vi "Match Multiple Geometric Patterns.vi"() -> ()   [LabVIEW 2014]
doc: "This example demonstrates how to perform multiple template geometric matching in NI Vision. First, three geometric matching templates are learned as a multiple geometric template. Next, the template is applied to a series of test images. This example uses color coded bounding boxes to display the location of geometric template matches and displays the number of instances of each geometric template match found in the test image."
uses:
  <vilib>/vision/Pattern Matching.llb/IMAQ Match Range Setting.ctl
  <vilib>/vision/NI_Vision_Development_Module.lvlib
panel:
  out "Hanger Matches":i32
  out "Plate Matches":i32
  out "Bracket Matches":i32
  in  "Delay (s.)":dbl(slide)=0.496 scale=0.0..2.0
  out "Image":T1(plugin-control)
  in  "Stop":bool
  in  "Hanger Color":u32(colorbox)=3381759
  in  "Plate Color":u32(colorbox)=6618880
  in  "Bracket Color":u32(colorbox)=16711680
  out "Hanger Template":T1(plugin-control)
  out "Plate Template":T1(plugin-control)
  out "Bracket Template":T1(plugin-control)
  # "Overview: Demonstrates how to use geometric matching to locate parts in an image.\nRequirements: NI Vision Development Module\nInstructions: Run the VI."
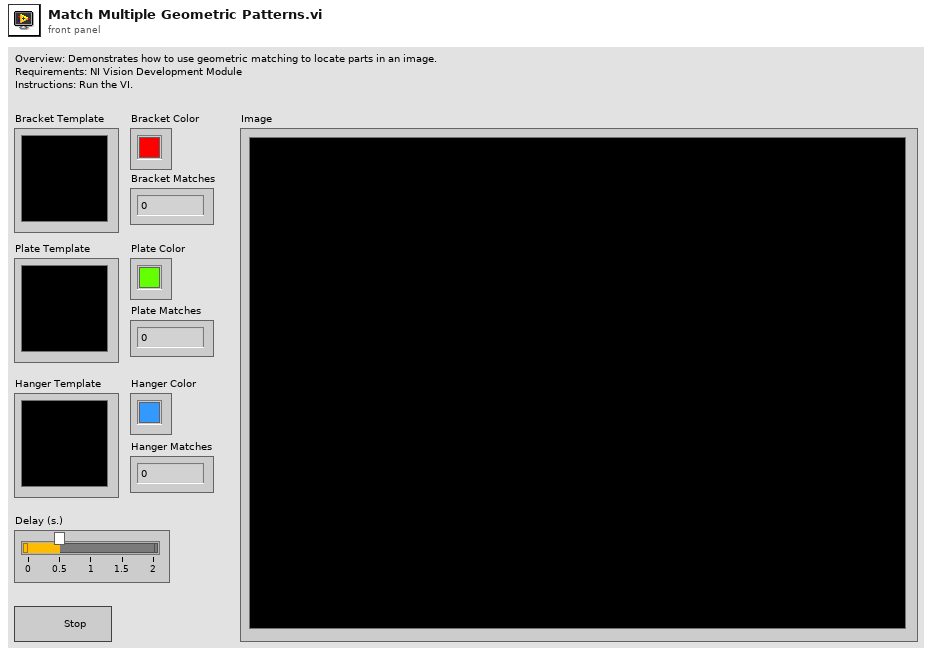
[diagram p1: front panel]
types:
  T1 = typedef "IMAQ Image.ctl" = refnum<image>
  T2 = typedef "IMAQ Match Range Setting.ctl" = cluster{"Match Constraints":u32, "Min":dbl, "Max":dbl}
  T3 = cluster{"Rotation":bool, "Scale":bool, "Occlusion":bool, "Reserved":bool, "Reserved":bool, "Reserved":bool}
  T4 = cluster{"Match Geometric Pattern Setup Data":string, "Number of Matches":i32, "Minimum Match Score":sgl}
  T5 = typedef "IMAQ GM Multiple Template.ctl" = refnum<k20>
  T6 = typedef "IMAQ GM Match Report.ctl" = cluster{"Position":cluster{"x":sgl, "y":sgl}, "Angle":sgl, "Scale":sgl, "Score":sgl, "Bounding Box":cluster{"x":sgl, "y":sgl}[], "Contrast Reversed":bool, "Occlusion %":sgl, "Template Target Curve Score":sgl, "Target Template Curve Score":sgl, "Correlation Score":sgl}
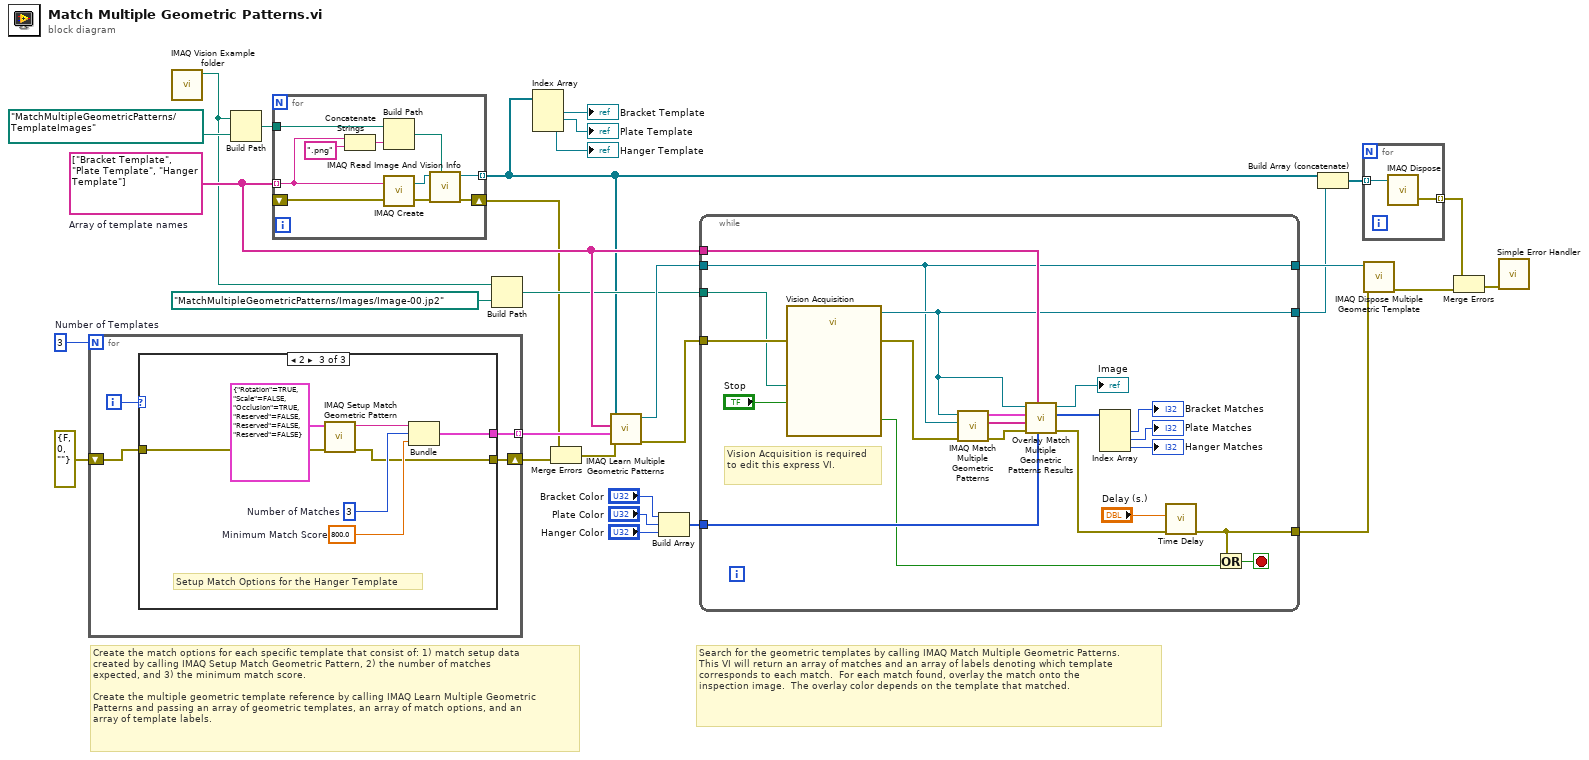
[diagram p0: block diagram]
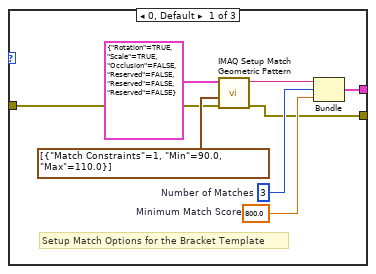
[diagram p2: hidden frame]
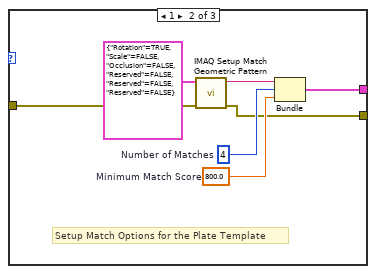
[diagram p3: hidden frame]
diagram:
  w15 = 3  # Number of Templates
  w21 = string[] ["Bracket Template", "Plate Template", "Hanger Template"]  # Array of template names
  # "Search for the geometric templates by calling IMAQ Match Multiple Geometric Patterns.\nThis VI will return an array of matches and an array of labels denoting which template\ncorresponds to each match.  For each match found, overlay the match onto the\ninspection image.  The overlay color depends on the template that matched."
  # "Create the match options for each specific template that consist of: 1) match setup data\ncreated by calling IMAQ Setup Match Geometric Pattern, 2) the number of matches \nexpected, and 3) the minimum match score.\n\nCreate the multiple geometric template reference by calling IMAQ Learn Multiple Geometric\nPatterns and passing an array of geometric templates, an array of match options, and an\narray of template labels."
  n1 = for {
    N: w15 -> [_]
    tunnel: [w33] -> w24 mode=indexing
    shift-right: [w31] -> w10
    shift-left: errorcluster {"status"=FALSE, "code"=0, "source"=""} ("error out") -> [w30]
    i -> [w32]
    n2 = case shown="2" w32 {
      tunnel: [w38 w45 w52] -> w33
      tunnel: [w35 w42 w49] -> w31
      tunnel: w30 -> [w34 w43 w50]
      frame 0, Default {
        w39 = sgl 800.0  # Minimum Match Score
        w40 = 3  # Number of Matches
        # "Setup Match Options for the Bracket Template"
        n3 = call "IMAQ Setup Match Geometric Pattern"("error in (no error)"=w34, "Range Settings"=T2[] [{"Match Constraints"=1, "Min"=90.0, "Max"=110.0}], "Match Mode"=T3 {"Rotation"=TRUE, "Scale"=TRUE, "Occlusion"=FALSE, "Reserved"=FALSE, "Reserved"=FALSE, "Reserved"=FALSE}) -> ("error out"=w35:errorcluster, "Match Geometric Pattern Setup Data"=w41:string)  [unwired: 7 in]
        n4 = Bundle("Match Geometric Pattern Setup Data"=w41, "Number of Matches"=w40, "Minimum Match Score"=w39) -> (w38:T4)  [unwired: 1 in]
      }
      frame 1 {
        w46 = sgl 800.0  # Minimum Match Score
        w47 = 4  # Number of Matches
        # "Setup Match Options for the Plate Template"
        n5 = call "IMAQ Setup Match Geometric Pattern"("error in (no error)"=w43, "Match Mode"=T3 {"Rotation"=TRUE, "Scale"=FALSE, "Occlusion"=FALSE, "Reserved"=FALSE, "Reserved"=FALSE, "Reserved"=FALSE}) -> ("error out"=w42:errorcluster, "Match Geometric Pattern Setup Data"=w48:string)  [unwired: 8 in]
        n6 = Bundle("Match Geometric Pattern Setup Data"=w48, "Number of Matches"=w47, "Minimum Match Score"=w46) -> (w45:T4)  [unwired: 1 in]
      }
      frame 2 {
        w53 = sgl 800.0  # Minimum Match Score
        w54 = 3  # Number of Matches
        # "Setup Match Options for the Hanger Template"
        n7 = call "IMAQ Setup Match Geometric Pattern"("error in (no error)"=w50, "Match Mode"=T3 {"Rotation"=TRUE, "Scale"=FALSE, "Occlusion"=TRUE, "Reserved"=FALSE, "Reserved"=FALSE, "Reserved"=FALSE}) -> ("error out"=w49:errorcluster, "Match Geometric Pattern Setup Data"=w55:string)  [unwired: 8 in]
        n8 = Bundle("Match Geometric Pattern Setup Data"=w55, "Number of Matches"=w54, "Minimum Match Score"=w53) -> (w52:T4)  [unwired: 1 in]
      }
    }
  }
  n9 = call "IMAQ Vision Example folder.vi"() -> ("Example Image Path"=w13:path)  [unwired: 11 in]
  n10 = Build Path(base path=w13, name or relative path=path "MatchMultipleGeometricPatterns/TemplateImages") -> (appended path=w25:path)
  n11 = for {
    tunnel: w21 -> [w61] mode=indexing
    tunnel: w25 -> [w65]
    tunnel: [w62] -> w5 mode=indexing
    shift-right: [w57] -> w9
    shift-left: _ -> [w56]
    n12 = Concatenate Strings(w61, ".png" ("string")) -> (w60:string)
    n13 = Build Path(base path=w65, name or relative path=w60) -> (appended path=w64:path)
    n14 = call "IMAQ Create"("Image Name"=w61, "error in (no error)"=w56) -> ("New Image"=w63:T1, "error out"=w58:errorcluster)  [unwired: 3 in]
    n15 = call "IMAQ Read Image And Vision Info"("File Path"=w64, "error in (no error)"=w58, "Image"=w63) -> ("error out"=w57:errorcluster, "Image Out"=w62:T1)  [unwired: 6 in, 1 out]
  }
  n16 = Build Path(base path=w13, name or relative path=path "MatchMultipleGeometricPatterns/Images/Image-00.jp2") -> (appended path=w12:path)
  n17 = Index Array(array=w5) -> (element #1=→"Bracket Template":T1, element #2=→"Plate Template":T1, element #3=→"Hanger Template":T1)  [unwired: 3 in]
  n18 = Merge Errors(w9, w10) -> (w8:errorcluster)
  n19 = call "IMAQ Learn Multiple Geometric Patterns"("error in (no error)"=w8, "Default Match Options"=w24, "Template Labels"=w21, "Template Images"=w5) -> ("error out"=w20:errorcluster, "Multiple Template (out)"=w23:T5)  [unwired: 6 in]
  n20 = Build Array("Bracket Color", "Plate Color", "Hanger Color") -> (w16:u32[])
  n21 = while {
    tunnel: w23 -> [w67]
    tunnel: w21 -> [w75]
    tunnel: [w67] -> w22
    tunnel: w20 -> [w80]
    tunnel: [w68] -> w6
    tunnel: w16 -> [w73]
    tunnel: w12 -> [w69]
    tunnel: [w66] -> w7
    stop <- w74 stop-if-true
    # "Vision Acquisition is required to edit this express VI."
    n22 = call "Vision Acquisition"("Image Path"=w69, "Stop (F)"="Stop", "error in"=w80) -> ("Image Out"=w68:T1, "Stopped"=w70:bool, "error out"=w72:errorcluster)  [unwired: 22 in]
    n23 = call "IMAQ Match Multiple Geometric Patterns"("error in (no error)"=w72, "Multiple Template"=w67, "Image"=w68) -> ("error out"=w78:errorcluster, "Matched Labels"=w76:string[], "Matches (pixel)"=w77:T6[])  [unwired: 5 in, 1 out]
    n24 = call "Overlay Match Multiple Geometric Patterns Results.vi"("Label Colors"=w73, "Learned Labels"=w75, "error in"=w78, "Match Labels"=w76, "Match Results"=w77, "Image"=w68) -> ("error out"=w71:errorcluster, "Number of Matches"=w79:i32[], "Image Out"=→"Image":T1)  [unwired: 3 in]
    n25 = Index Array(array=w79) -> (element #1=→"Bracket Matches":i32, element #2=→"Plate Matches":i32, element #3=→"Hanger Matches":i32)  [unwired: 3 in]
    n26 = call "Time Delay"("error in (no error)"=w71, "Delay Time (s)"="Delay (s.)") -> ("error out"=w66:errorcluster)  [unwired: 9 in]
    n27 = Or(x=w66, y=w70) -> (x .or. y?=w74:bool)
  }
  n28 = Build Array (concatenate)(w5, w6) -> (w4:T1[])
  n29 = for {
    tunnel: w4 -> [w88] mode=indexing
    tunnel: [w87] -> w2 mode=indexing
    n30 = call "IMAQ Dispose"("Image"=w88) -> ("error out"=w87:errorcluster)  [unwired: 5 in]
  }
  n31 = call "IMAQ Dispose Multiple Geometric Template"("error in (no error)"=w7, "Multiple Template"=w22) -> ("error out"=w3:errorcluster)  [unwired: 9 in]
  n32 = Merge Errors(w2, w3) -> (w1:errorcluster)
  n33 = call <vilib>:"Simple Error Handler.vi"("error in (no error)"=w1) -> ()  [unwired: 4 in, 5 out]
